vi "Checkers Settings.vi"() -> ()   [LabVIEW 2014]
uses:
  Game Info Global Variable.vi
panel:
  out "Boolean 4":bool
  in  "Boolean 3":bool
  out "Boolean 2":bool
  in  "Boolean":bool
  in  "P2 Blue Text Color:":i32
  in  "P2 Green Text Color:":i32
  in  "P2 Red Text Color:":i32
  in  "P2 Blue Color:":i32
  in  "P2 Green Color:":i32
  in  "P2 Red Color:":i32
  in  "P1 Blue Text Color:":i32
  in  "P1 Green Text Color:":i32
  in  "P1 Red Text Color:":i32
  in  "P1 Blue Color:":i32
  in  "P1 Green Color:":i32
  in  "P1 Red Color:":i32
  in  "Blue:":string="255"
  in  "Green:":string="255"
  in  "Red:":string="255"
  in  "Blue:":string="0"
  in  "Green:":string="0"
  in  "Red:":string="0"
  in  "Main Menu":bool
  in  "Apply Changes":bool
  out "new picture 4":picture
  out "new picture 2":picture
  out "new picture":picture
  out "new picture 3":picture
  out "King:":picture
  out "Piece:":picture
  # "SETTINGS:"
  # "Game Appearance:"
  # "Player 1 Piece/King Color:"
  # "Turn Marker:"
  # "Piece:"
  # "King:"
  # "Player 1 King Text Color:"
  # "Player 2 Piece/King Color:"
  # "Piece:"
  # "King:"
  # "Turn Marker:"
  # "Player 2 King Text Color:"
  # "Board Square Color 1:"
  # "Board Square 1:"
  # "Board Square 1:"
  # "Board Square Color 2:"
  # "Optional Rules:"
  # "Own-Man Jump Rule:"
  # "Force Capture Rule:"
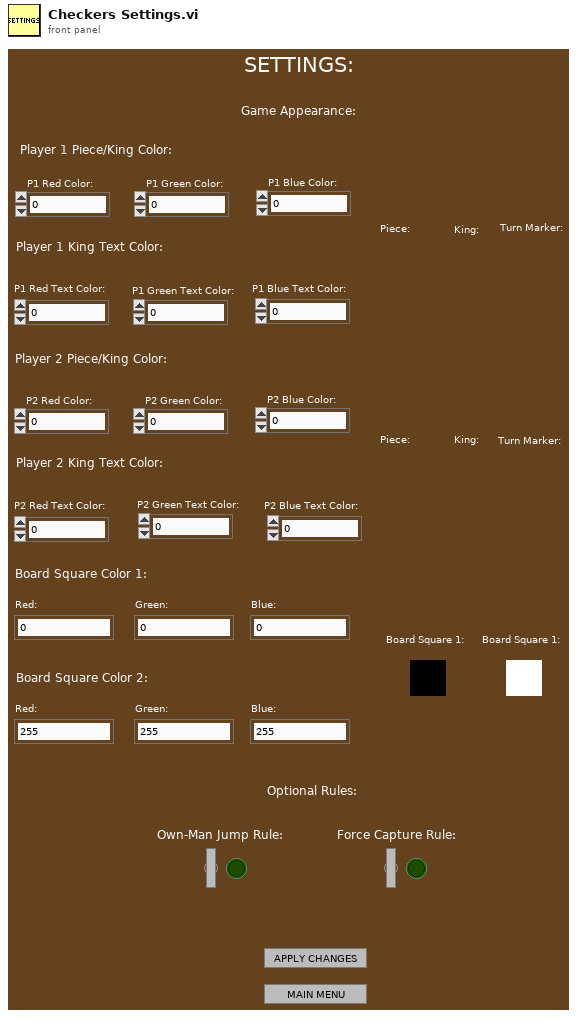
[diagram p1: front panel]
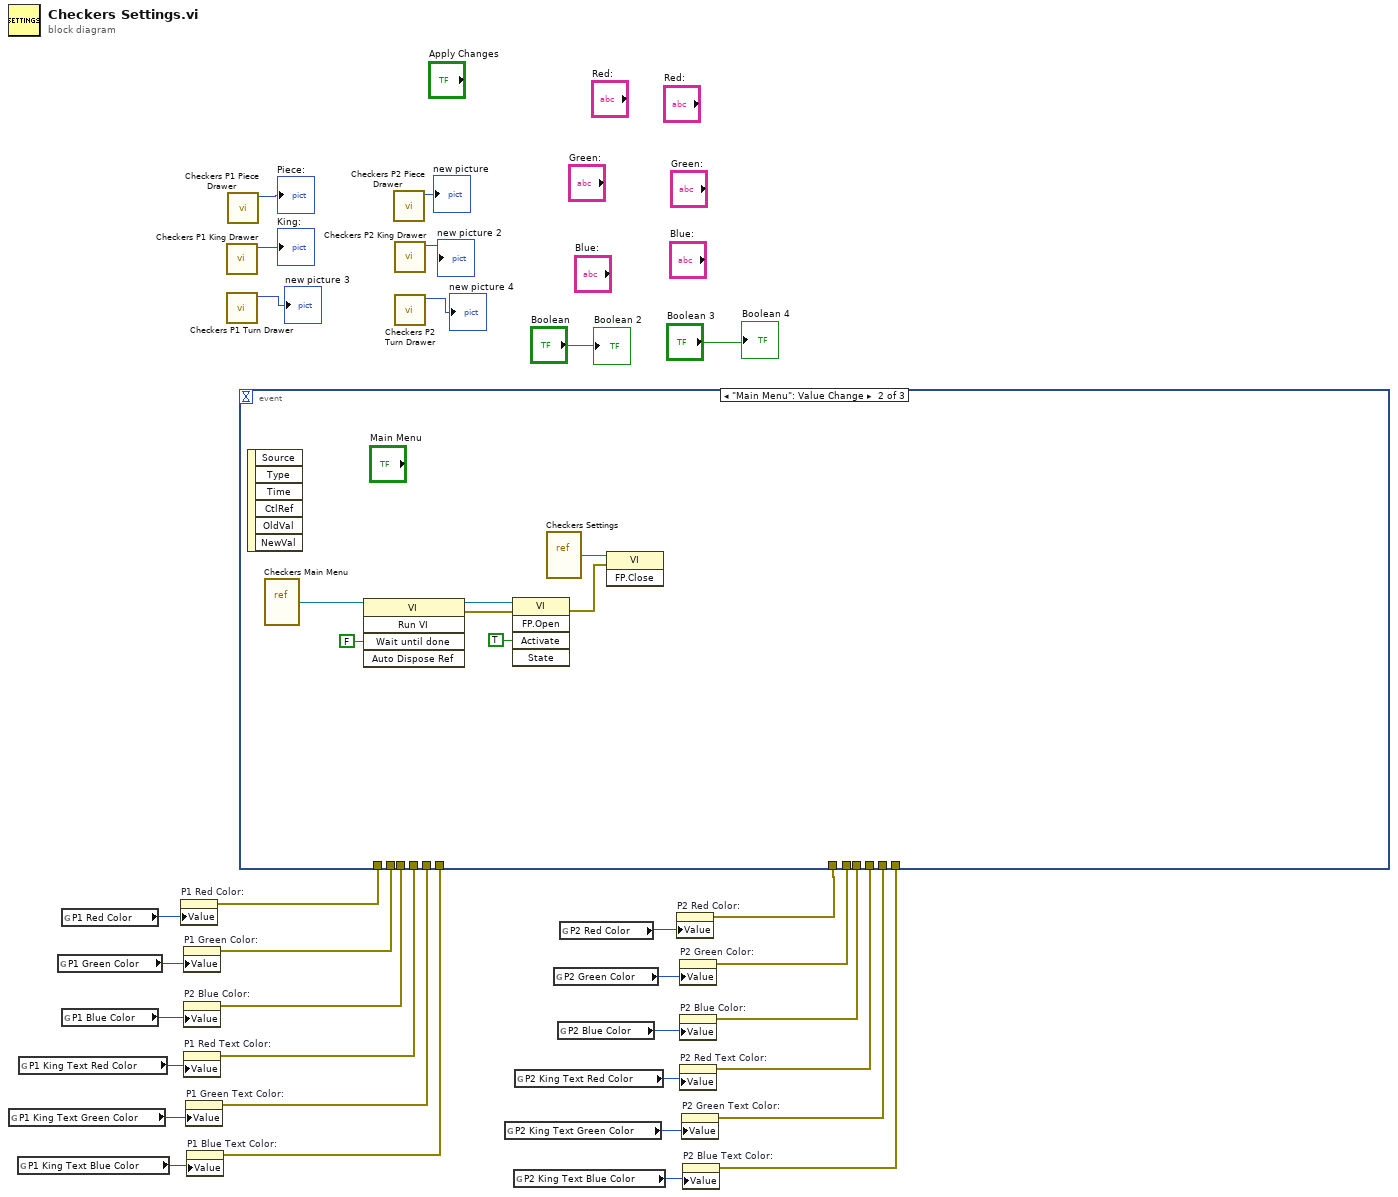
[diagram p0: block diagram]
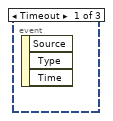
[diagram p2: hidden frame]
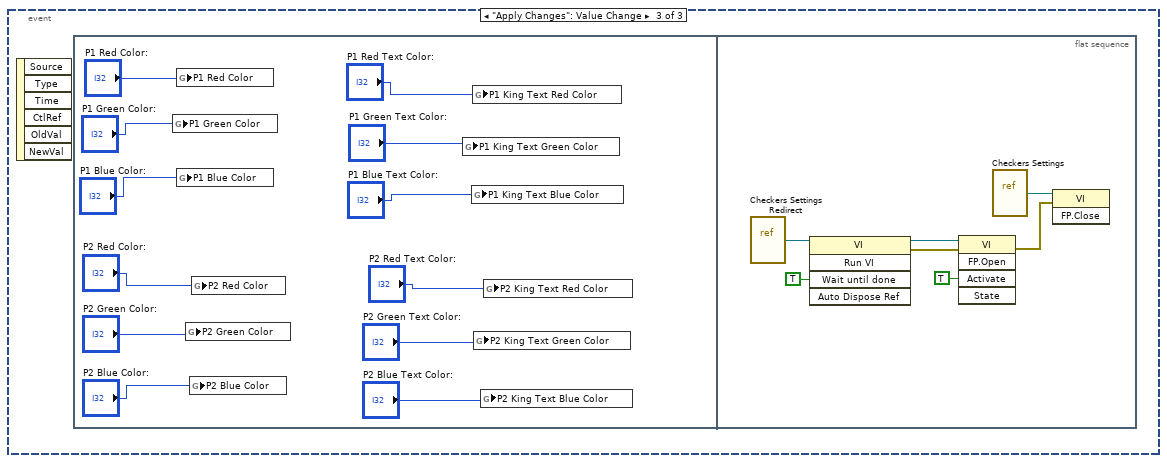
[diagram p3: hidden frame]
diagram:
  n1 = global read "Game Info Global Variable.vi" "P1 King Text Green Color"() -> (w19:i32)
  n2 = global read "Game Info Global Variable.vi" "P1 King Text Blue Color"() -> (w18:i32)
  n3 = global read "Game Info Global Variable.vi" "P1 King Text Red Color"() -> (w20:i32)
  n4 = global read "Game Info Global Variable.vi" "P1 Green Color"() -> (w24:i32)
  n5 = global read "Game Info Global Variable.vi" "P1 Red Color"() -> (w26:i32)
  n6 = global read "Game Info Global Variable.vi" "P1 Blue Color"() -> (w22:i32)
  n7 = property on="P1 Red Color:" class="DigNum (strict)"("Value"=w26) -> (error out=w25:errorcluster)  [unwired: 2 in, 1 out]
  n8 = property on="P1 Green Color:" class="DigNum (strict)"("Value"=w24) -> (error out=w23:errorcluster)  [unwired: 2 in, 1 out]
  n9 = property on="P2 Blue Color:" class="DigNum (strict)"("Value"=w22) -> (error out=w21:errorcluster)  [unwired: 2 in, 1 out]
  n10 = property on="P1 Red Text Color:" class="DigNum (strict)"("Value"=w20) -> (error out=w17:errorcluster)  [unwired: 2 in, 1 out]
  n11 = property on="P1 Green Text Color:" class="DigNum (strict)"("Value"=w19) -> (error out=w16:errorcluster)  [unwired: 2 in, 1 out]
  n12 = property on="P1 Blue Text Color:" class="DigNum (strict)"("Value"=w18) -> (error out=w15:errorcluster)  [unwired: 2 in, 1 out]
  n13 = call "Checkers P1 King Drawer.vi"() -> ("new picture"=→"King:":picture)  [unwired: 11 in]
  n14 = call "Checkers P1 Turn Drawer.vi"() -> ("new picture"=→"new picture 3":picture)  [unwired: 11 in]
  n15 = call "Checkers P1 Piece Drawer.vi"() -> ("new picture"=→"Piece:":picture)  [unwired: 11 in]
  n16 = call "Checkers P2 Piece Drawer.vi"() -> ("new picture"=→"new picture":picture)  [unwired: 11 in]
  n17 = call "Checkers P2 King Drawer.vi"() -> ("new picture"=→"new picture 2":picture)  [unwired: 11 in]
  n18 = call "Checkers P2 Turn Drawer.vi"() -> ("new picture"=→"new picture 4":picture)  [unwired: 11 in]
  n19 = global read "Game Info Global Variable.vi" "P2 King Text Green Color"() -> (w13:i32)
  n20 = global read "Game Info Global Variable.vi" "P2 King Text Blue Color"() -> (w14:i32)
  n21 = global read "Game Info Global Variable.vi" "P2 King Text Red Color"() -> (w12:i32)
  n22 = global read "Game Info Global Variable.vi" "P2 Green Color"() -> (w10:i32)
  n23 = global read "Game Info Global Variable.vi" "P2 Blue Color"() -> (w11:i32)
  n24 = global read "Game Info Global Variable.vi" "P2 Red Color"() -> (w9:i32)
  n25 = property on="P2 Red Color:" class="DigNum (strict)"("Value"=w9) -> (error out=w8:errorcluster)  [unwired: 2 in, 1 out]
  n26 = property on="P2 Green Color:" class="DigNum (strict)"("Value"=w10) -> (error out=w7:errorcluster)  [unwired: 2 in, 1 out]
  n27 = property on="P2 Blue Color:" class="DigNum (strict)"("Value"=w11) -> (error out=w6:errorcluster)  [unwired: 2 in, 1 out]
  n28 = property on="P2 Red Text Color:" class="DigNum (strict)"("Value"=w12) -> (error out=w5:errorcluster)  [unwired: 2 in, 1 out]
  n29 = property on="P2 Green Text Color:" class="DigNum (strict)"("Value"=w13) -> (error out=w4:errorcluster)  [unwired: 2 in, 1 out]
  n30 = property on="P2 Blue Text Color:" class="DigNum (strict)"("Value"=w14) -> (error out=w3:errorcluster)  [unwired: 2 in, 1 out]
  n31 = event shown="[1] \"Main Menu\": Value Change" {
    selector: _ -> [_ _ _]
    dyn-events: _ -> [_ _ _]
    timeout: _ -> [_ _ _]
    tunnel: w25 -> [_ _ _]
    tunnel: w23 -> [_ _ _]
    tunnel: w21 -> [_ _ _]
    tunnel: w17 -> [_ _ _]
    tunnel: w16 -> [_ _ _]
    tunnel: w15 -> [_ _ _]
    tunnel: w8 -> [_ _ _]
    tunnel: w7 -> [_ _ _]
    tunnel: w6 -> [_ _ _]
    tunnel: w5 -> [_ _ _]
    tunnel: w4 -> [_ _ _]
    tunnel: w3 -> [_ _ _]
    event Timeout {
      n32 = event-data() -> ()  [unwired: 1 in, 3 out]
    }
    event "Main Menu": Value Change {
      n33 = event-data() -> ()  [unwired: 1 in, 6 out]
      n34 = vi-ref "Checkers Main Menu.vi"() -> (w39:refnum<vi>)
      n35 = invoke class="VI" method="Run VI"(reference=w39, "Wait until done"=FALSE ("Wait Until Done")) -> (reference out=w38:refnum<vi>, error out=w37:errorcluster)  [unwired: 3 in, 3 out]
      n36 = invoke class="VI" method="FP.Open"(reference=w38, error in=w37, "Activate"=TRUE ("Activate?")) -> (error out=w33:errorcluster)  [unwired: 2 in, 4 out]
      n37 = vi-ref "Checkers Settings.vi"() -> (w34:refnum<vi>)
      n38 = invoke class="VI" method="FP.Close"(reference=w34, error in=w33) -> ()  [unwired: 1 in, 3 out]
    }
    event "Apply Changes": Value Change {
      n39 = event-data() -> ()  [unwired: 1 in, 6 out]
      n40 = flat-sequence {
        frame #0 {
          n41 = global write "Game Info Global Variable.vi" "P1 Green Color"("P1 Green Color:") -> ()
          n42 = global write "Game Info Global Variable.vi" "P1 Red Color"("P1 Red Color:") -> ()
          n43 = global write "Game Info Global Variable.vi" "P1 Blue Color"("P1 Blue Color:") -> ()
          n44 = global write "Game Info Global Variable.vi" "P2 Green Color"("P2 Green Color:") -> ()
          n45 = global write "Game Info Global Variable.vi" "P2 Blue Color"("P2 Blue Color:") -> ()
          n46 = global write "Game Info Global Variable.vi" "P2 Red Color"("P2 Red Color:") -> ()
          n47 = global write "Game Info Global Variable.vi" "P1 King Text Green Color"("P1 Green Text Color:") -> ()
          n48 = global write "Game Info Global Variable.vi" "P1 King Text Blue Color"("P1 Blue Text Color:") -> ()
          n49 = global write "Game Info Global Variable.vi" "P1 King Text Red Color"("P1 Red Text Color:") -> ()
          n50 = global write "Game Info Global Variable.vi" "P2 King Text Green Color"("P2 Green Text Color:") -> ()
          n51 = global write "Game Info Global Variable.vi" "P2 King Text Blue Color"("P2 Blue Text Color:") -> ()
          n52 = global write "Game Info Global Variable.vi" "P2 King Text Red Color"("P2 Red Text Color:") -> ()
        }
        frame #1 {
          n53 = vi-ref "Checkers Settings Redirect.vi"() -> (w58:refnum<vi>)
          n54 = invoke class="VI" method="Run VI"(reference=w58, "Wait until done"=TRUE ("Wait Until Done")) -> (reference out=w57:refnum<vi>, error out=w56:errorcluster)  [unwired: 3 in, 3 out]
          n55 = invoke class="VI" method="FP.Open"(reference=w57, error in=w56, "Activate"=TRUE ("Activate?")) -> (error out=w53:errorcluster)  [unwired: 2 in, 4 out]
          n56 = vi-ref "Checkers Settings.vi"() -> (w52:refnum<vi>)
          n57 = invoke class="VI" method="FP.Close"(reference=w52, error in=w53) -> ()  [unwired: 1 in, 3 out]
        }
      }
    }
  }
  "Boolean 2" <- "Boolean"
  "Boolean 4" <- "Boolean 3"
